vi "DistSignal.vi"(0 "Offset AC":dbl caption="Offset", 5 "Frequency":dbl=50.0, 7 "Amplitude":dbl=5.0, 9 "Phase":dbl, 11 "Offset DC":dbl=5.0 caption="Offset") -> (4 "Waveform Chart":dynamicdata(graph))   [LabVIEW 2021]
uses:
  <vilib>/express/express shared/transition.llb/Dynamic To Waveform Array.vi
  <vilib>/express/express signal manip/GetorSetDDTAttributes/Set DDT Attributes/SetT0.vi
  <vilib>/express/express signal manip/GetorSetDDTAttributes/Set DDT Attributes/sub Set StartTimeStamp.vi
  <vilib>/express/express shared/transition.llb/Waveform Array To Dynamic.vi
  <vilib>/express/express signal manip/GetorSetDDTAttributes/Set DDT Attributes/Set DDT Properties.xnode
  <vilib>/express/express signal manip/GetorSetDDTAttributes/Set DDT Attributes/Set DDT Attributes.lvlib
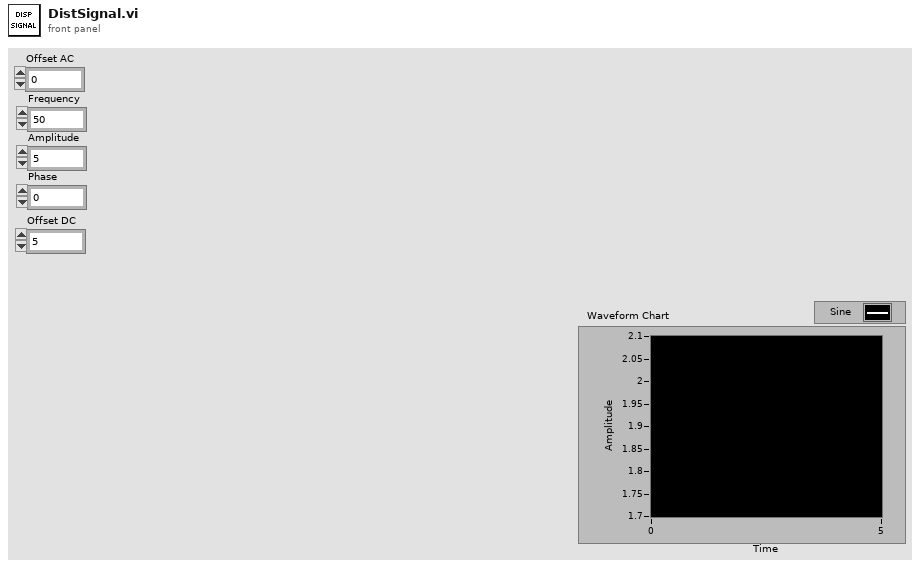
[diagram p1: front panel]
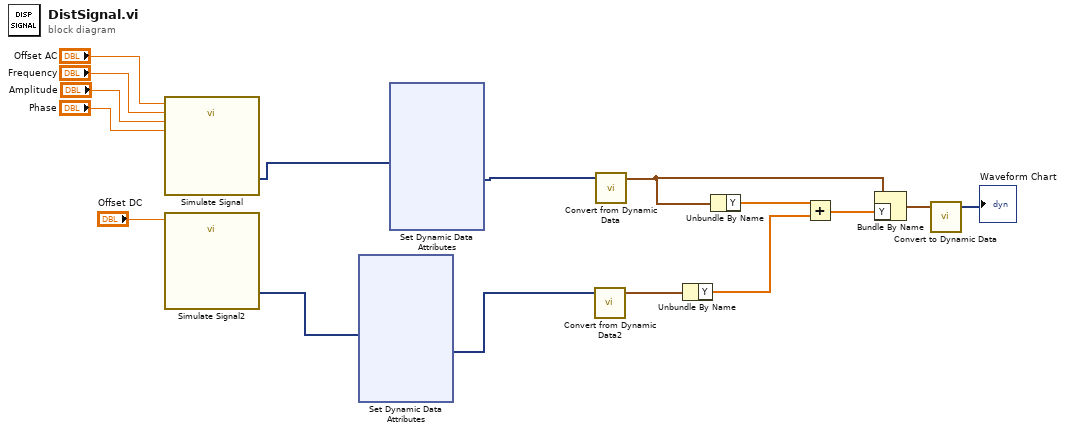
[diagram p0: block diagram]
diagram:
  n1 = call "Simulate Signal"("Offset"="Offset AC", "Frequency"="Frequency", "Amplitude"="Amplitude", "Phase"="Phase") -> ("Sine"=w3:dynamicdata)  [unwired: 10 in, 1 out]
  n2 = call "Simulate Signal2"("Offset"="Offset DC") -> ("DC"=w16:dynamicdata)  [unwired: 13 in, 1 out]
  n3 = xnode "Set Dynamic Data Attributes"("Signals In"=w16) -> ("Signals Out"=w1:dynamicdata)  [unwired: 3 in, 1 out]
  n4 = xnode "Set Dynamic Data Attributes"("Signals In"=w3) -> ("Signals Out"=w2:dynamicdata)  [unwired: 3 in, 1 out]
  n5 = call "Convert from Dynamic Data2"("Dynamic Data Type"=w1) -> ("Waveform"=w15:waveform(dbl))  [unwired: 3 in]
  n6 = call "Convert from Dynamic Data"("Dynamic Data Type"=w2) -> ("Waveform"=w12:waveform(dbl))  [unwired: 3 in]
  n7 = Unbundle By Name(w15) -> ("Y"=w13:dbl[])
  n8 = Unbundle By Name ("Get Waveform Components")(w12) -> ("Y"=w14:dbl[])
  n9 = Add(x=w14, y=w13) -> (x+y=w11:dbl[])
  n10 = Bundle By Name ("Build Waveform")(cluster=w12, "Y"=w11) -> (w10:waveform(dbl))
  n11 = call "Convert to Dynamic Data"("Waveform"=w10) -> ("Dynamic Data Type"=→"Waveform Chart":dynamicdata)  [unwired: 3 in]
